vi "Configure.vi"(8 "error in":errorcluster, 10 "name":string, 11 "CRDS in":refnum<class "CRDS.lvclass">) -> (0 "error out":errorcluster, 3 "CRDS out":refnum<class "CRDS.lvclass">)   [LabVIEW 2017, in "CRDS Lib.lvlib" / "CRDS.lvclass"]
doc: "Configure the instrument class. If there is no config file specified, an error"
uses:
  CRDS.lvclass
  Z:/sw_repo/For Builds/Reusable/Instrument/Instrument.lvclass
  Data/Main/CRDS Data.lvclass
  Z:/sw_repo/For Builds/Reusable/Data/Data.lvclass
  General/Math/Fit Exponential Class/Children/LRS/LRS.lvclass
  Z:/sw_repo/For Builds/Reusable/General/Math/Fit Exponential Class/Fit Exponential.lvclass
  General/Math/Fit Exponential Class/Fit Exponential.lvclass/Fit Exponential.ctl
  Instrument/Instrument.lvclass/Instrument.ctl
  Session APIs/File Access/Config Data/Config Data.lvclass/Config Data.ctl
  Data/Cell/CRDS Cell Data.lvclass
  Data/Data.lvclass/Data.ctl
  Data/Cell/CRDS Cell Data.lvclass/CRDS Cell Data.ctl
  Cell/CRDS Cell.lvclass/CRDS Cell.ctl
  Data/Write Data ID.vi
  Data/Cell/Write Ncell.vi
  Data/Cell/Write Write RD_.vi
  Cell/Write ExpFit.vi
  Cell/Write Data.vi
  General/Math/Fit Exponential Class/Write Get A_B.vi
  Instrument/Read Cfg Session.vi
  Instrument/Read ExtCom.vi
  Session APIs/File Access/Config Data/Accessors/Read Ref.vi
  Instrument/Write Data OK_.vi
  Instrument/Write Data.vi
  Read Cells.vi
  <vilib>/Utility/config.llb/Read Key (I32).vi
  <vilib>/Utility/config.llb/Read Key (Boolean).vi
  Session APIs/File Access/Config Data/Read Array/Read DBL Array.vi
  Session APIs/File Access/Config Data/Read Array/Read String Array.vi
  General/Atmospheric/Atmospheric Constants.vi
  Cell/Write lambda.vi
  Cell/Write optTimeConst.vi
  Data/Main/Write CellData.vi
  Write Cells.vi
  Instrument/Instrument.lvclass
  Cell/CRDS Cell.lvclass
  Session APIs/File Access/Config Data/Config Data.lvclass
  <vilib>/Utility/config.llb/NI_LVConfig.lvlib
  General/Atmospheric/Atmospheric Library.lvlib
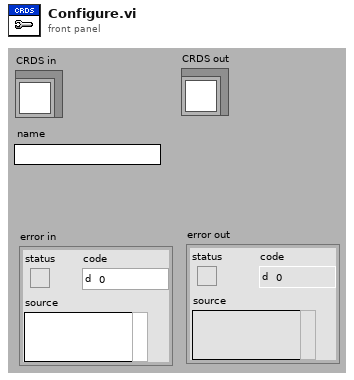
[diagram p1: front panel]
types:
  T1 = cluster{"tag":string, "section":string, "data":variant}
  T2 = typedef "NI_LVConfig.lvlib/Config Data RefNum.ctl" = refnum<k1>
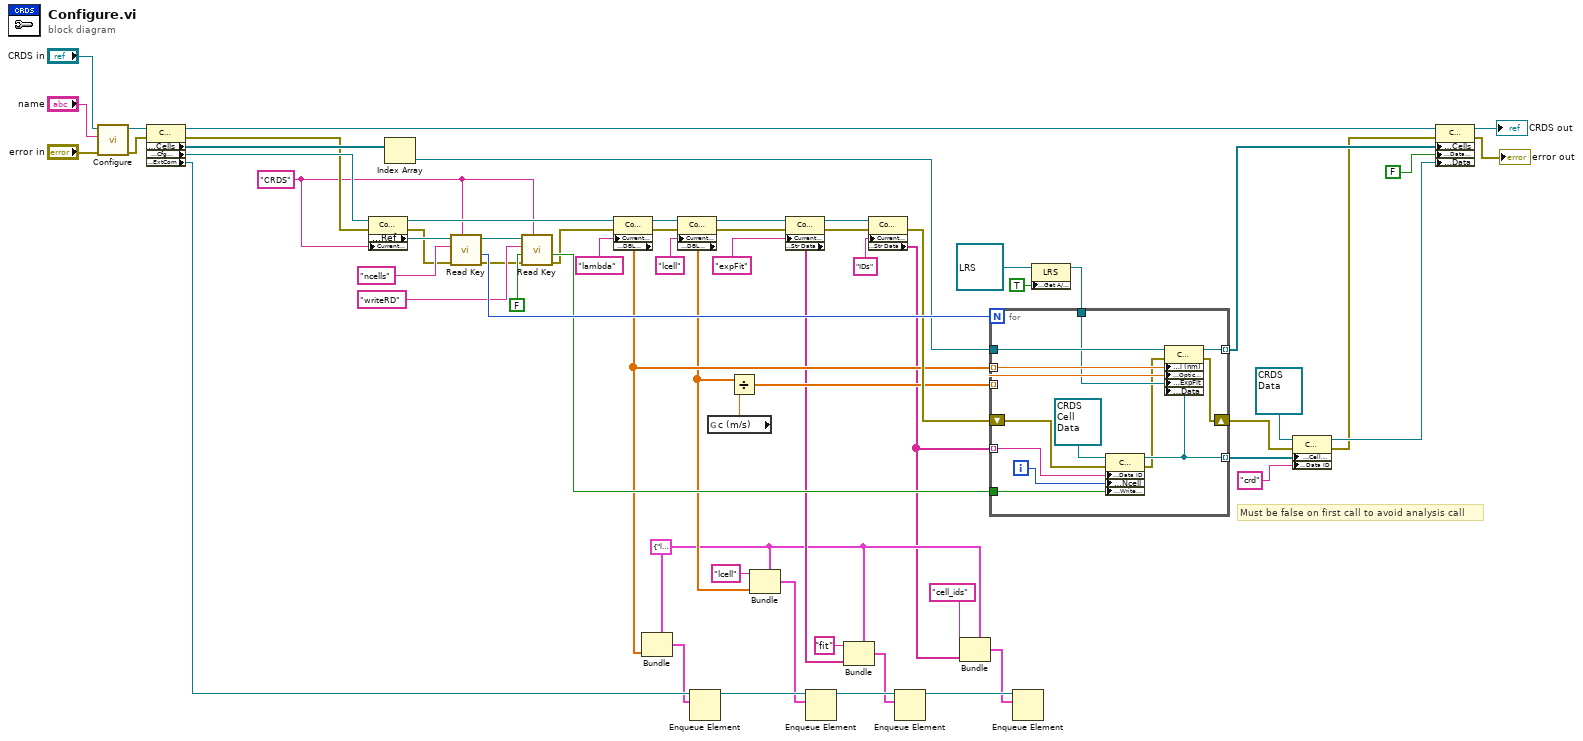
[diagram p0: block diagram]
diagram:
  w10 = T1 {"tag"="lambda", "section"="crd", "data"=variant} ("element")
  w26 = "CRDS" ("section")
  # "Must be false on first call to avoid analysis call"
  n1 = call-parent "Configure.vi"("error in"="error in", "name"="name", "Instrument in"="CRDS in") -> ("error out"=w34:errorcluster, "Instrument out"=w61:refnum<class "CRDS.lvclass">)  [unwired: 7 in]
  n2 = property class="CRDS"(reference=w61, error in=w34) -> (reference out=w49:refnum<class "CRDS.lvclass">, error out=w31:errorcluster, "Data Access:Cells"=w32:refnum<class "CRDS Cell.lvclass">[], "Accessors:Cfg Session"=w33:refnum<data-value>, "Accessors:ExtCom"=w16:refnum<queue>)
  n3 = property class="Config Data"(reference=w33, error in=w31, "Current Section"=w26) -> (reference out=w59:refnum<data-value>, error out=w27:errorcluster, "Accessors:Ref"=w28:T2)
  n4 = Index Array(array=w32) -> (element=w51:refnum<class "CRDS Cell.lvclass">)  [unwired: 1 in]
  n5 = call-poly <vilib>:"Read Key.vi"("section"=w26, "error in (no error)"=w27, "key"="ncells", "refnum"=w28) -> ("error out"=w29:errorcluster, "value"=w52:i32, "refnum out"=w30:T2)  [unwired: 4 in, 1 out]
  n6 = call-poly <vilib>:"Read Key.vi"("section"=w26, "error in (no error)"=w29, "default value"=FALSE, "key"="writeRD", "refnum"=w30) -> ("error out"=w25:errorcluster, "value"=w38:bool)  [unwired: 3 in, 2 out]
  n7 = property class="Config Data"(reference=w59, error in=w25, "Current Key"="lambda") -> (reference out=w57:refnum<data-value>, error out=w56:errorcluster, "Read Array Data:DBL Data"=w15:dbl[])
  n8 = Bundle(cluster=w10, "data"=w15) -> (w7:T1)  [unwired: 2 in]
  n9 = property class="Config Data"(reference=w57, error in=w56, "Current Key"="lcell") -> (reference out=w55:refnum<data-value>, error out=w54:errorcluster, "Read Array Data:DBL Data"=w13:dbl[])
  n10 = Enqueue Element(queue=w16, element=w7) -> (queue out=w6:refnum<queue>)  [unwired: 2 in, 2 out]
  n11 = global read "Atmospheric Constants.vi" "c (m/s)"() -> (w18:dbl)
  n12 = Divide(x=w13, y=w18) -> (x/y=w17:dbl[])
  n13 = Bundle(cluster=w10, "tag"="lcell", "data"=w13) -> (w5:T1)  [unwired: 1 in]
  n14 = property class="Config Data"(reference=w55, error in=w54, "Current Key"="expFit") -> (reference out=w22:refnum<data-value>, error out=w20:errorcluster, "Read Array Data:Str Data"=w12:string[])
  n15 = Enqueue Element(queue=w6, element=w5) -> (queue out=w4:refnum<queue>)  [unwired: 2 in, 2 out]
  n16 = Bundle(cluster=w10, "tag"="fit", "data"=w12) -> (w3:T1)  [unwired: 1 in]
  n17 = property class="Config Data"(reference=w22, error in=w20, "Current Key"="IDs") -> (error out=w19:errorcluster, "Read Array Data:Str Data"=w9:string[])  [unwired: 1 out]
  n18 = Enqueue Element(queue=w4, element=w3) -> (queue out=w2:refnum<queue>)  [unwired: 2 in, 2 out]
  n19 = Bundle(cluster=w10, "tag"="cell_ids", "data"=w9) -> (w1:T1)  [unwired: 1 in]
  n20 = Enqueue Element(queue=w2, element=w1) -> ()  [unwired: 2 in, 3 out]
  n21 = property class="LRS"(reference=refnum<class "LRS.lvclass"> refnum ("Exponential Fit Lib:LRS"), "Accessors:Get A/B?"=TRUE ("Get A/B?")) -> (reference out=w35:refnum<class "LRS.lvclass">)  [unwired: 1 in, 1 out]
  n22 = for {
    N: w52 -> [_]
    tunnel: w51 -> [w77]
    tunnel: w17 -> [w76] mode=indexing
    tunnel: w15 -> [w75] mode=indexing
    tunnel: [w73] -> w48 mode=indexing
    tunnel: [w70] -> w43 mode=indexing
    tunnel: w35 -> [w72]
    tunnel: w38 -> [w68]
    shift-right: [w74] -> w24
    shift-left: w19 -> [w67]
    tunnel: w9 -> [w65] mode=indexing
    i -> [w69]
    n23 = property class="CRDS Cell"(reference=refnum<class "CRDS Cell Data.lvclass"> refnum ("CRDS Cell"), error in=w67, "Accessors:Data ID"=w65, "Data Access:Ncell"=w69, "Data Access:Write RD_"=w68) -> (reference out=w70:refnum<class "CRDS Cell Data.lvclass">, error out=w66:errorcluster)
    n24 = property class="CRDS Cell"(reference=w77, error in=w66, "Accessors:l (nm)"=w75, "Accessors:Optical Time Constant"=w76, "Accessors:ExpFit"=w72, "Accessors:Data"=w70) -> (reference out=w73:refnum<class "CRDS Cell.lvclass">, error out=w74:errorcluster)
  }
  n25 = property class="CRDS"(reference=refnum<class "CRDS Data.lvclass"> refnum ("CRDS"), error in=w24, "Accessors:Cell Data"=w43, "Accessors:Data ID"="crd" ("Data ID")) -> (reference out=w42:refnum<class "CRDS Data.lvclass">, error out=w23:errorcluster)
  n26 = property class="CRDS"(reference=w49, error in=w23, "Data Access:Cells"=w48, "Accessors:Data OK_"=FALSE ("Data Ready?"), "Accessors:Data"=w42) -> (reference out=→"CRDS out":refnum<class "CRDS.lvclass">, error out=→"error out":errorcluster)
